vi "fICHERO2.vi"() -> ()   [LabVIEW 2020]
uses:
  <vilib>/numeric/Random Number (Range) DBL.vi
  <vilib>/Utility/file.llb/Write Delimited Spreadsheet (DBL).vi
panel:
  in  "String":string
  in  "Stop Button":bool
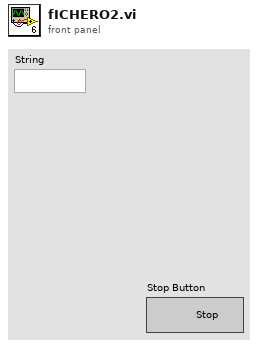
[diagram p1: front panel]
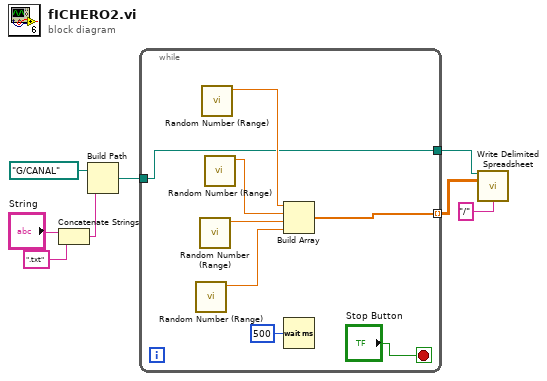
[diagram p0: block diagram]
diagram:
  n1 = Concatenate Strings("String", ".txt" ("string")) -> (w5:string)
  n2 = Build Path(base path=path "G:/CANAL", name or relative path=w5) -> (appended path=w4:path)
  n3 = while {
    tunnel: [w11] -> w2 mode=indexing
    tunnel: w4 -> [w10]
    tunnel: [w10] -> w3
    stop <- "Stop Button" stop-if-true
    n4 = call-poly <vilib>:"Random Number (Range).vi"() -> ("number"=w9:dbl)  [unwired: 11 in]
    n5 = call-poly <vilib>:"Random Number (Range).vi"() -> ("number"=w12:dbl)  [unwired: 11 in]
    n6 = call-poly <vilib>:"Random Number (Range).vi"() -> ("number"=w14:dbl)  [unwired: 11 in]
    n7 = call-poly <vilib>:"Random Number (Range).vi"() -> ("number"=w13:dbl)  [unwired: 11 in]
    n8 = Build Array(w14, w13, w12, w9) -> (w11:dbl[])
    n9 = Wait (ms)(milliseconds to wait=u32 500) -> ()  [unwired: 1 out]
  }
  n10 = call-poly <vilib>:"Write Delimited Spreadsheet.vi"("file path (dialog if empty)"=w3, "2D data"=w2, "delimiter (\\t)"="/" ("delimiter (\\t)")) -> ()  [unwired: 11 in, 2 out]
